vi "VoltageMeasure.vi"(8 "Error In":errorcluster, 11 "DMMIn":refnum<class "DMM.lvclass">) -> (0 "Error Out":errorcluster, 2 "Measurement":dbl, 3 "DMMOut":refnum<class "DMM.lvclass">)   [LabVIEW 2019, in "DMM.lvclass"]
uses:
  DMM.lvclass
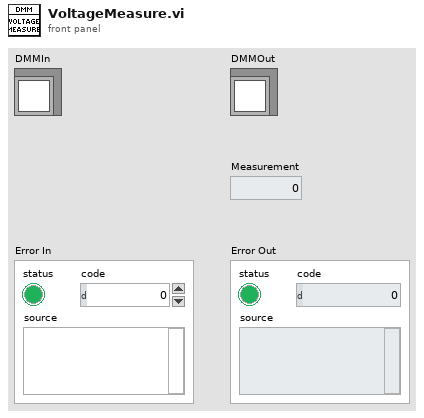
[diagram p1: front panel]
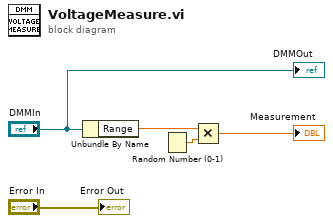
[diagram p0: block diagram]
diagram:
  n1 = Unbundle By Name("DMMIn") -> ("Range"=w3:dbl)
  n2 = Random Number (0-1)() -> (number: 0 to 1=w2:dbl)
  n3 = Multiply(x=w3, y=w2) -> (x*y=→"Measurement":dbl)
  "DMMOut" <- "DMMIn"
  "Error Out" <- "Error In"
